vi "Write Boolean.vi"(9 "Boolean":bool, 11 "Boolean Event in":refnum<class "Boolean Event.lvclass">) -> (3 "Boolean Event out":refnum<class "Boolean Event.lvclass">)   [LabVIEW 2016, in "Boolean Event.lvclass"]
uses:
  Boolean Event.lvclass
  Boolean Event.lvclass/Boolean Event.ctl
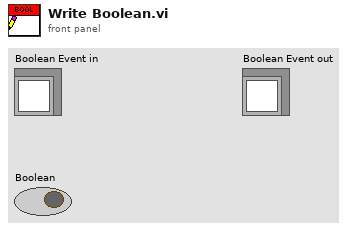
[diagram p1: front panel]
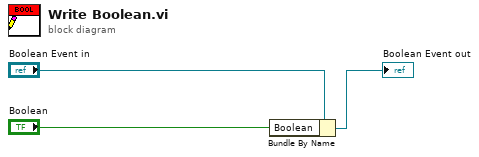
[diagram p0: block diagram]
diagram:
  n1 = Bundle By Name(cluster="Boolean Event in", "Boolean"="Boolean") -> (→"Boolean Event out":refnum<class "Boolean Event.lvclass">)
